vi "testpractice.vi"() -> ()   [LabVIEW 2016]
uses:
  <vilib>/measure/NI_MABase.lvlib
  <vilib>/Analysis/3filter.llb/Filter Passband Type.ctl
  <vilib>/Analysis/NI_AALBase.lvlib
panel:
  out "output waveform 3":waveform(dbl)(graph)
  out "output waveform 2":waveform(dbl)(graph)
  in  "order":i32=2
  in  "low cutoff freq: fl":dbl=0.12500000000000006 format="%0.4f"
  out "Waveform":waveform(dbl)(graph)
  in  "frequency":dbl=10.0 format="%0.2p"
  out "size(s)":i32
  in  "Numeric":dbl format="%#_13g"
  out "output waveform":waveform(dbl)(graph)
  in  "Low Value":i32
  in  "High Value":i32
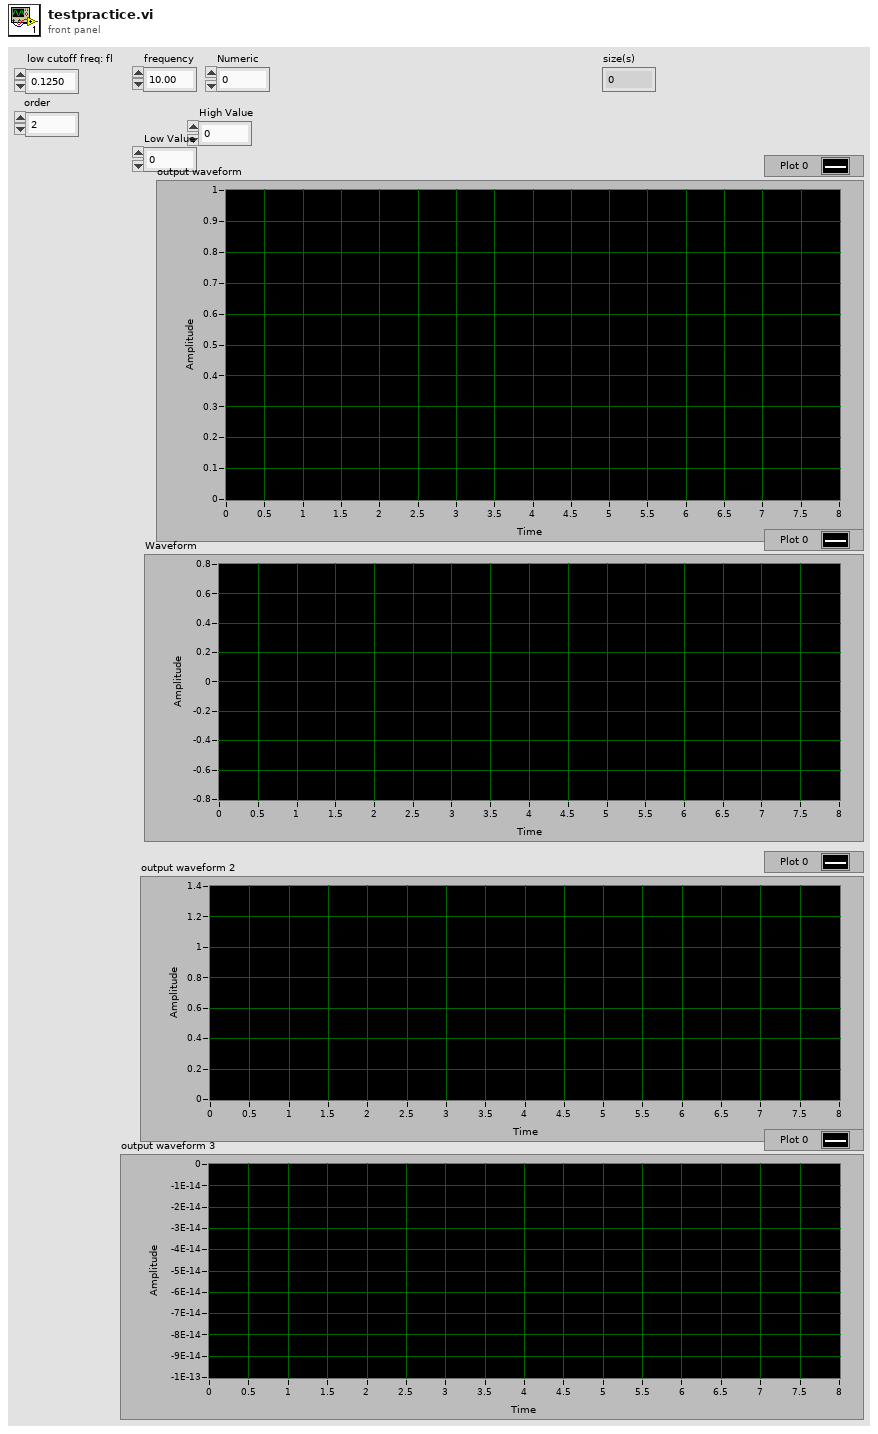
[diagram p1: front panel]
types:
  T1 = typedef "NI_AALBase.lvlib/Filter Passband Type.ctl" = enum32{"Lowpass", "Highpass", "Bandpass", "Bandstop"}
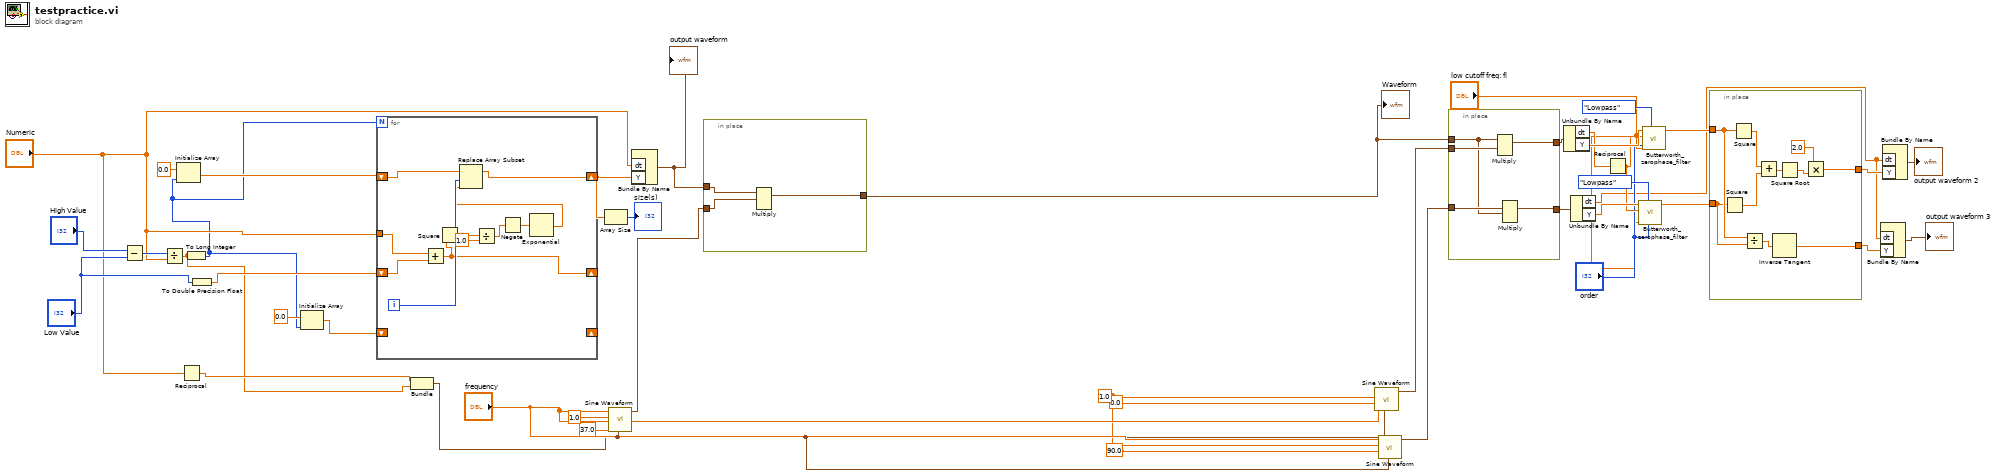
[diagram p0: block diagram]
diagram:
  w25 = 1.0 ("amplitude")
  n1 = Subtract(x="High Value", y="Low Value") -> (x-y=w41:i32)
  n2 = Divide(x=w41, y="Numeric") -> (x/y=w29:dbl)
  n3 = Reciprocal(x="Numeric") -> (1/x=w30:dbl)
  n4 = To Long Integer(number=w29) -> (32bit integer=w2:i32)
  n5 = Initialize Array(0.0 ("element"), w2) -> (w39:dbl[])
  n6 = To Double Precision Float(number="Low Value") -> (double precision float=w37:dbl)
  n7 = Initialize Array(0.0 ("element"), w2) -> (w1:dbl[])
  n8 = for {
    N: w2 -> [_]
    shift-right: [w54] -> w36
    shift-left: w39 -> [w53]
    tunnel: "Numeric" -> [w52]
    shift-right: [w48] -> _
    shift-left: w37 -> [w51]
    shift-right: _ -> [_]
    shift-left: w1 -> [_]
    i -> [w50]
    n9 = Add(x=w52, y=w51) -> (x+y=w48:dbl)
    n10 = Square(x=w48) -> (x^2=w47:dbl)
    n11 = Divide(x=w47, y=1.0) -> (x/y=w45:dbl)
    n12 = Negate(x=w45) -> (-x=w44:dbl)
    n13 = Exponential(1:w44) -> (0:w49:dbl)
    n14 = Replace Array Subset(array=w53, new element=w49, index=w50) -> (w54:dbl[])
  }
  n15 = Bundle(w30, w29) -> (w7:cluster{dbl, dbl})  [unwired: 1 in]
  n16 = Array Size(array=w36) -> (size(s)=→"size(s)":i32)
  n17 = call <vilib>:"Sine Waveform.vi"("sampling info"=w7, "phase"=37.0, "amplitude"=1.0, "frequency"="frequency") -> ("signal out"=w34:waveform(dbl))  [unwired: 6 in, 1 out]
  n18 = Bundle By Name("dt"="Numeric", "Y"=w36) -> (w33:waveform(dbl))  [unwired: 1 in]
  "output waveform" <- w33
  n19 = in-place {
    in-place-border: w34 -> [w57]
    in-place-border: w33 -> [w56]
    in-place-border: [w55] -> w28
    n20 = Multiply(1:w57, 2:w56) -> (0:w55:waveform(dbl))  [unwired: 1 in, 1 out]
  }
  "Waveform" <- w28
  n21 = call <vilib>:"Sine Waveform.vi"("sampling info"=w7, "phase"=0.0, "amplitude"=w25, "frequency"="frequency") -> ("signal out"=w27:waveform(dbl))  [unwired: 6 in, 1 out]
  n22 = call <vilib>:"Sine Waveform.vi"("sampling info"=w7, "phase"=90.0, "amplitude"=w25, "frequency"="frequency") -> ("signal out"=w22:waveform(dbl))  [unwired: 6 in, 1 out]
  n23 = in-place {
    in-place-border: w28 -> [w60]
    in-place-border: w27 -> [w62]
    in-place-border: w22 -> [w61]
    in-place-border: [w59] -> w21
    in-place-border: [w58] -> w19
    n24 = Multiply(1:w62, 2:w60) -> (0:w59:waveform(dbl))  [unwired: 1 in, 1 out]
    n25 = Multiply(1:w60, 2:w61) -> (0:w58:waveform(dbl))  [unwired: 1 in, 1 out]
  }
  n26 = Unbundle By Name(w21) -> ("dt"=w17:dbl, "Y"=w20:dbl[])
  n27 = Unbundle By Name(w19) -> ("dt"=w5:dbl, "Y"=w18:dbl[])
  n28 = Reciprocal(x=w17) -> (1/x=w16:dbl)
  n29 = call "Butterworth_zerophase_filter.vi"("order"="order", "filter type"=Filter_Passband_Type."Lowpass", "low cutoff freq: fl"="low cutoff freq: fl", "sampling freq: fs"=w16, "X"=w18) -> ("Filtered X"=w11:dbl[])  [unwired: 5 in, 1 out]
  n30 = call "Butterworth_zerophase_filter.vi"("order"="order", "filter type"=Filter_Passband_Type."Lowpass", "low cutoff freq: fl"="low cutoff freq: fl", "sampling freq: fs"=w16, "X"=w20) -> ("Filtered X"=w12:dbl[])  [unwired: 5 in, 1 out]
  n31 = in-place {
    in-place-border: w12 -> [w65]
    in-place-border: w11 -> [w64]
    in-place-border: [w67] -> w10
    in-place-border: [w63] -> w6
    n32 = Square(x=w64) -> (x^2=w71:dbl[])
    n33 = Square(x=w65) -> (x^2=w72:dbl[])
    n34 = Divide(x=w65, y=w64) -> (x/y=w66:dbl[])
    n35 = Add(x=w72, y=w71) -> (x+y=w70:dbl[])
    n36 = Inverse Tangent(1:w66) -> (0:w63:dbl[])
    n37 = Square Root(x=w70) -> (sqrt(x)=w69:dbl[])
    n38 = Multiply(x=2.0, y=w69) -> (x*y=w67:dbl[])
  }
  n39 = Bundle By Name("dt"=w5, "Y"=w6) -> (→"output waveform 3":waveform(dbl))  [unwired: 1 in]
  n40 = Bundle By Name("dt"=w5, "Y"=w10) -> (→"output waveform 2":waveform(dbl))  [unwired: 1 in]
